vi "isCache.vi"(11 "ConfigManager.Cache in":refnum<class "ConfigManager.Cache.lvclass">) -> (2 "isCache?":bool, 3 "ConfigManager.Cache out":refnum<class "ConfigManager.Cache.lvclass">)   [LabVIEW 2013, in "SMOConfig.lvlib" / "ConfigManager.Cache.lvclass"]
uses:
  ConfigManager.Cache.lvclass
  ConfigManager.Cache.lvclass/ConfigManager.Cache.ctl
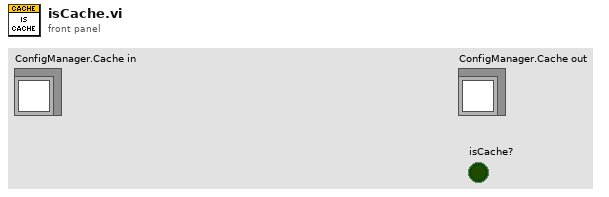
[diagram p1: front panel]
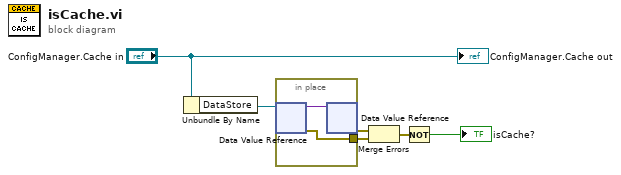
[diagram p0: block diagram]
diagram:
  n1 = Unbundle By Name("ConfigManager.Cache in") -> ("DataStore"=w5:refnum<data-value>)
  n2 = in-place {
    in-place-border: [w7] -> w3
    n3 = in-place-dvr #1(w5) -> (w8:variant, w7:errorcluster)
    n4 = in-place-dvr #1(w8) -> (w4:errorcluster)  [unwired: 1 out]
  }
  n5 = Merge Errors(w4, w3) -> (w2:errorcluster)
  n6 = Not(x=w2) -> (.not. x?=→"isCache?":bool)
  "ConfigManager.Cache out" <- "ConfigManager.Cache in"
